vi "Get DAQ Metadata.vi"(10 "Channel":string, 11 "Task":refnum<k21>) -> (2 "Metadata":T1)   [LabVIEW 2013]
uses:
  XControls/Sensor Metadata.ctl
  <resource>/objmgr/daqmx.rc
panel:
  out "AI.MeasType":i32(ring)=10322 items=["Voltage"=10322, "Voltage RMS"=10350, "Current"=10134, "Current RMS"=10351, "More:Voltage:Custom with Excitation"=10323, "More:Bridge (V/V)"=15908, "Frequency"=10181, "Resistance"=10278, "Temperature:Thermocouple"=10303, "Temperature:Thermistor"=10302, "Temperature:RTD"=10301, "Temperature:Built-in Sensor"=10311, "Strain Gage"=10300, "Rosette Strain Gage"=15980, "Position:LVDT"=10352, "Position:RVDT"=10353, "Position:Eddy Current Proximity Probe"=14835, "Accelerometer"=10356, "Velocity:IEPE Sensor"=15966, "Force:Bridge"=15899, "Force:IEPE Sensor"=15895, "Pressure:Bridge"=15902, "Sound Pressure:Microphone"=10354, "Torque:Bridge"=15905, "TEDS Sensor"=12531]
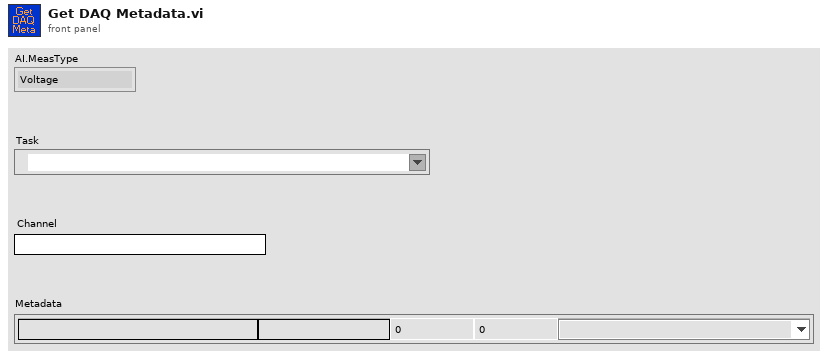
[diagram p1: front panel]
types:
  T1 = typedef "Sensor Metadata.ctl" = cluster{"Name":string, "Units":string, "Multiplier":dbl, "Excitation":u16, "Sensitivity":dbl}
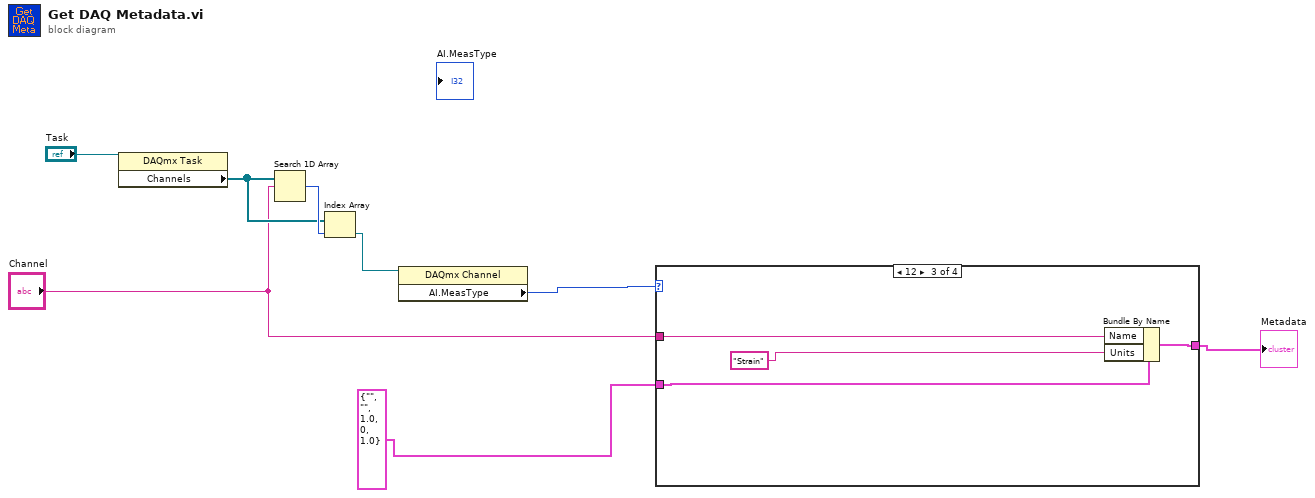
[diagram p0: block diagram]
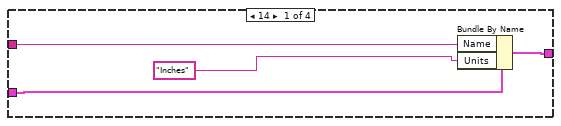
[diagram p2: hidden frame]
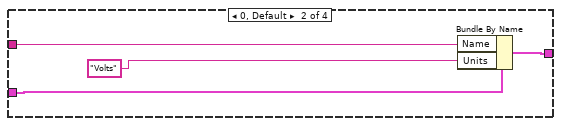
[diagram p3: hidden frame]
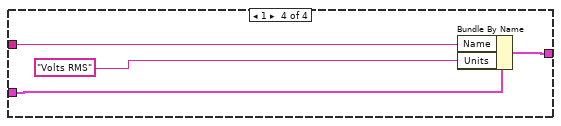
[diagram p4: hidden frame]
diagram:
  n1 = property class="DAQmx Task"(reference="Task") -> ("Channels"=w6:refnum<k21>[])  [unwired: 1 in, 2 out]
  n2 = Search 1D Array(1D array=w6, element="Channel") -> (index of element=w7:i32)  [unwired: 1 in]
  n3 = Index Array(array=w6, index=w7) -> (element=w5:refnum<k21>)
  n4 = property class="DAQmx Channel"(reference=w5) -> ("AI.MeasType"=w1:i32)  [unwired: 1 in, 2 out]
  n5 = case shown="12" w1 {
    tunnel: T1 {"Name"="", "Units"="", "Multiplier"=1.0, "Excitation"=0, "Sensitivity"=1.0} ("Metadata") -> [w10 w15 w19 w23]
    tunnel: "Channel" -> [w12 w16 w20 w24]
    tunnel: [w9 w14 w18 w22] -> w2
    frame 14 {
      n6 = Bundle By Name(cluster=w10, "Name"=w12, "Units"="Inches" ("element")) -> (w9:T1)
    }
    frame 0, Default {
      n7 = Bundle By Name(cluster=w15, "Name"=w16, "Units"="Volts" ("element")) -> (w14:T1)
    }
    frame 12 {
      n8 = Bundle By Name(cluster=w19, "Name"=w20, "Units"="Strain" ("element")) -> (w18:T1)
    }
    frame 1 {
      n9 = Bundle By Name(cluster=w23, "Name"=w24, "Units"="Volts RMS" ("element")) -> (w22:T1)
    }
  }
  "Metadata" <- w2
